vi "Port Number and Machine Name.vi"(0 "LV DEV.lvclass":refnum<class "LV DEV.lvclass">, 5 "PID":string, 11 "error in (no error)":errorcluster) -> (4 "LV DEV.lvclass":refnum<class "LV DEV.lvclass">, 6 "Machine Name":string, 8 "Port Number":u16, 15 "error out":errorcluster)   [LabVIEW 2016, in "LV DEV.lvclass"]
uses:
  LV DEV.lvclass
  <vilib>/regexp/Match Regular Expression.xnode
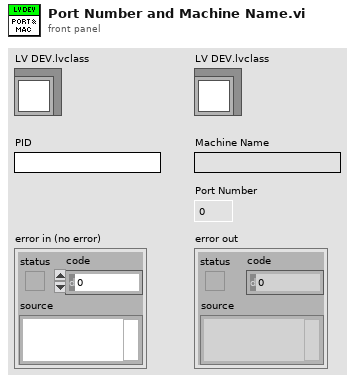
[diagram p1: front panel]
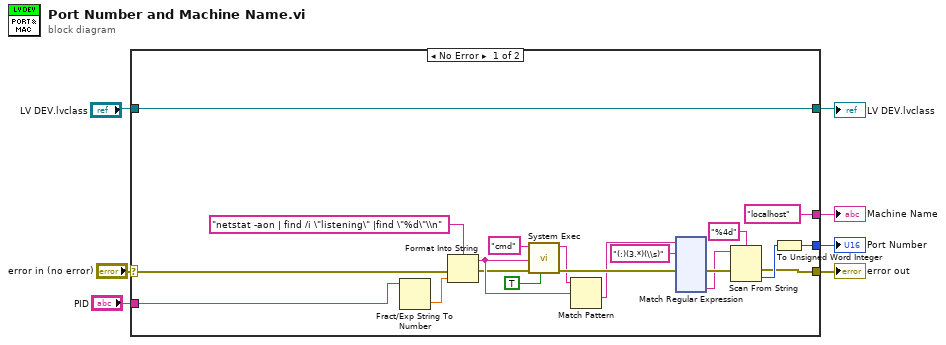
[diagram p0: block diagram]
diagram:
  n1 = case shown="No Error" "error in (no error)" {
    selector: "error in (no error)" -> [w13 w146]
    tunnel: [w12 w146] -> w6
    tunnel: [w27 w145] -> w1
    tunnel: "LV DEV.lvclass" -> [w27 w145]
    tunnel: "PID" -> [w11 _]
    tunnel: ["localhost" _] -> w4
    tunnel: [w9 _] -> w3
    frame No Error {
      n2 = Fract/Exp String To Number(string=w11) -> (number=w26:dbl)  [unwired: 3 in, 1 out]
      n3 = Format Into String(format string="netstat -aon | find /i \"listening\" |find \"%d\"\\n" ("standard input"), error in=w13, w26) -> (resulting string=w18:string, error out=w16:errorcluster)  [unwired: 1 in]
      n4 = call <vilib>:"System Exec.vi"("run minimized? (F)"=TRUE, "error in (no error)"=w16, "standard input"=w18, "command line"="cmd") -> ("error out"=w21:errorcluster, "standard output"=w17:string)  [unwired: 4 in, 2 out]
      n5 = Match Pattern(string=w17, regular expression=w18) -> (after substring=w19:string)  [unwired: 1 in, 3 out]
      n6 = xnode "Match Regular Expression"("input string"=w19, "regular expression"="(:)(3.*)(\\s)", "error in"=w21) -> ("error out"=w25:errorcluster, "submatch 2"=w22:string)  [unwired: 3 in, 5 out]
      n7 = Scan From String(format string="%4d", input string=w22, error in=w25) -> (error out=w12:errorcluster, output 1=w24:i32)  [unwired: 2 in, 2 out]
      n8 = To Unsigned Word Integer(number=w24) -> (unsigned 16bit integer=w9:u16)
    }
    frame Error {
    }
  }
  "error out" <- w6
  "Port Number" <- w3
  "Machine Name" <- w4
  "LV DEV.lvclass" <- w1
